vi "Controller Test Bench (6).vi"() -> ()   [LabVIEW 2022 SP3]
uses:
  <vilib>/sound2/lvsound2.llb/Sound Data Format.ctl
  <vilib>/Utility/error.llb/DialogType.ctl
  <vilib>/sound2/lvsound2.llb/Sampling Mode.ctl
  <vilib>/Analysis/4window.llb/windowTd.ctl
  <vilib>/DAQmx/read.llb/DAQmx Read (Analog 1D Wfm NChan NSamp).vi
  <vilib>/DAQmx/write.llb/DAQmx Write (Analog 1D DBL 1Chan NSamp).vi
  <vilib>/DAQmx/create/channels.llb/DAQmx Create Channel (AI-Acceleration-Accelerometer).vi
  <vilib>/DAQmx/create/channels.llb/DAQmx Create Channel (AO-Voltage-Basic).vi
  <vilib>/DAQmx/configure/timing.llb/DAQmx Timing (Sample Clock).vi
  <vilib>/DAQmx/miscellaneous.llb/DAQmx Fill In Error Info.vi
  <vilib>/measure/maspectr.llb/FFT Spectrum (Mag-Phase) for N Chan.vi
  <vilib>/DAQmx/configure/task.llb/DAQmx Configure Logging (TDMS).vi
  <vilib>/sound2/lvsound2.llb/Sound Output Set Volume (Single).vi
  <vilib>/sound2/lvsound2.llb/Sound Output Write (DBL Single).vi
  <resource>/objmgr/daqmx.rc
  <vilib>/Analysis/NI_AALPro.lvlib
  <vilib>/measure/NI_MAPro.lvlib
panel:
  out "number of samples written per channel":u32
  in  "Active Control":bool
  in  "Output Noise":bool
  in  "Log Data":bool
  out "Phase 2":cluster{"f0":dbl, "df":dbl, "phase":dbl[]}[](graph)
  out "Mag 2":cluster{"f0":dbl, "df":dbl, "magnitude":dbl[]}[](graph)
  in  "Show FFT":bool
  in  "Save FFT":bool
  in  "Start Acquisition":bool
  in  "Stop":bool
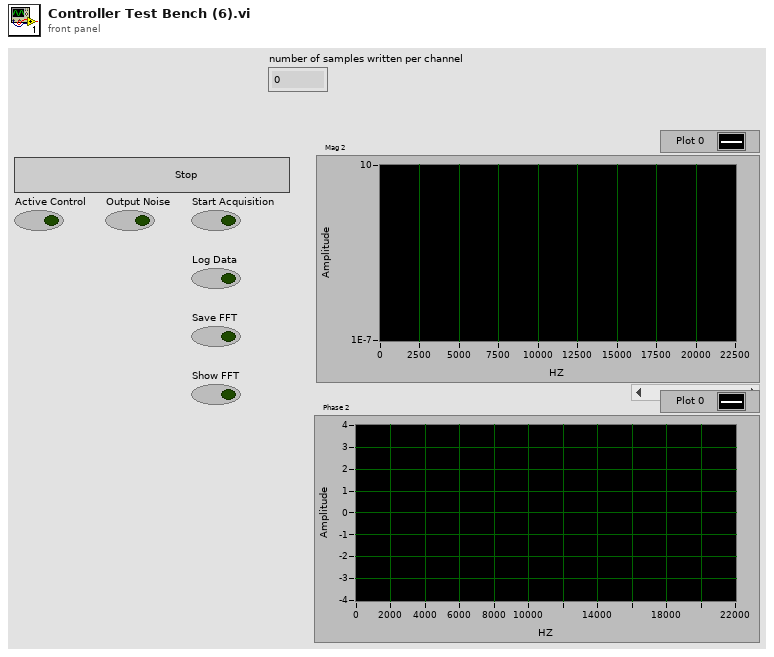
[diagram p1: front panel]
types:
  T1 = typedef "Sampling Mode.ctl" = i32
  T2 = typedef "DialogType.ctl" = u16
  T3 = typedef "Sound Data Format.ctl" = cluster{"sample rate (S/s)":dbl, "number of channels":i32, "bits per sample":i32}
  T4 = typedef "Sound Output Task ID.ctl" = u32
  T5 = typedef "NI_AALPro.lvlib/windowTd.ctl" = u32
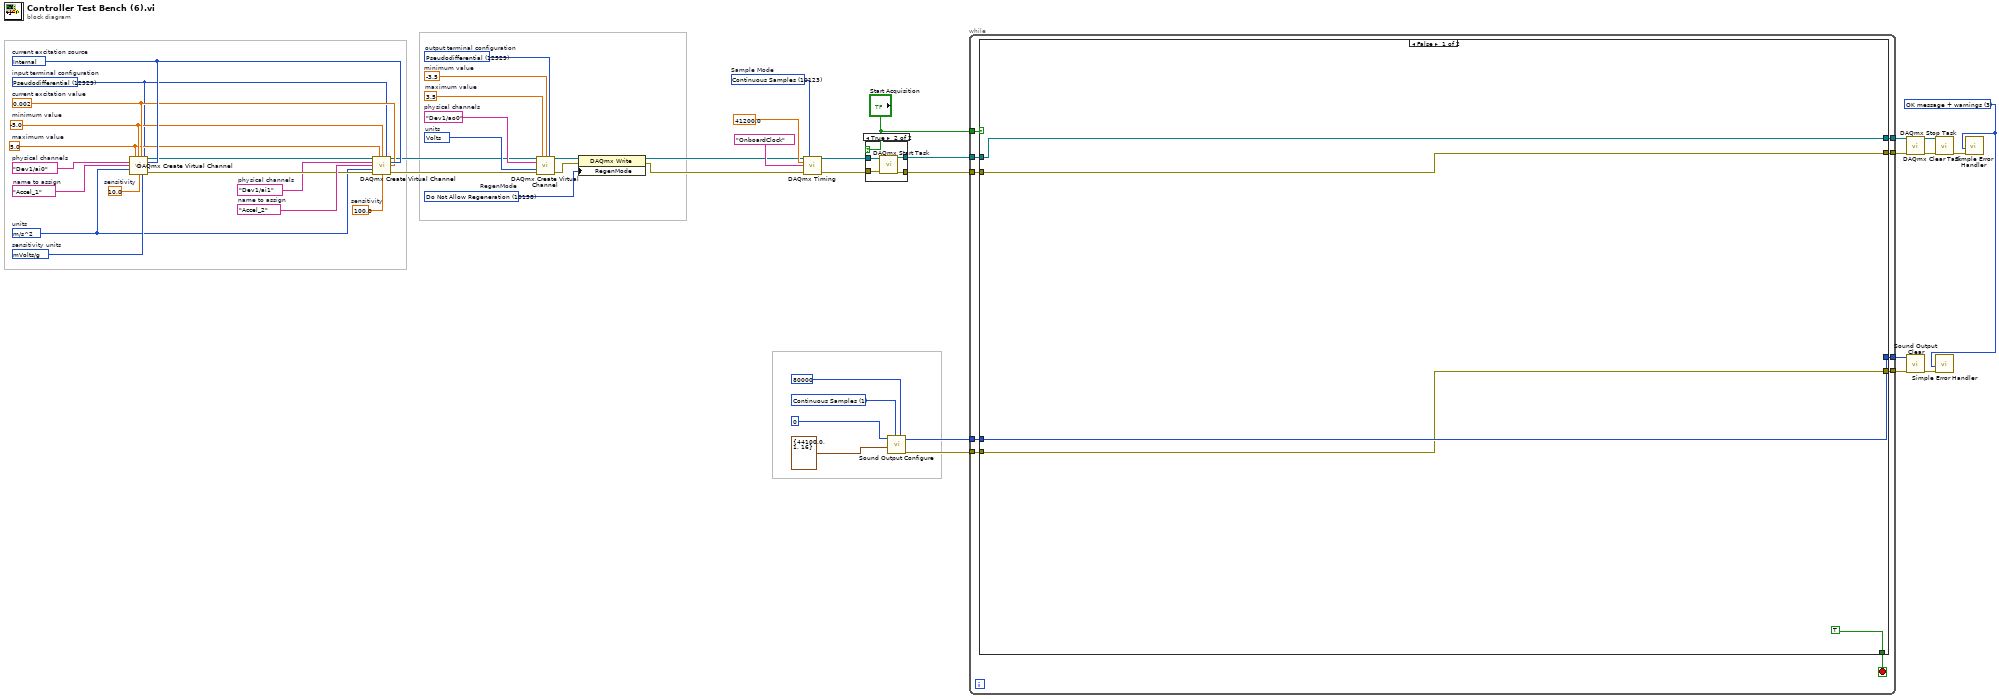
[diagram p0: block diagram]
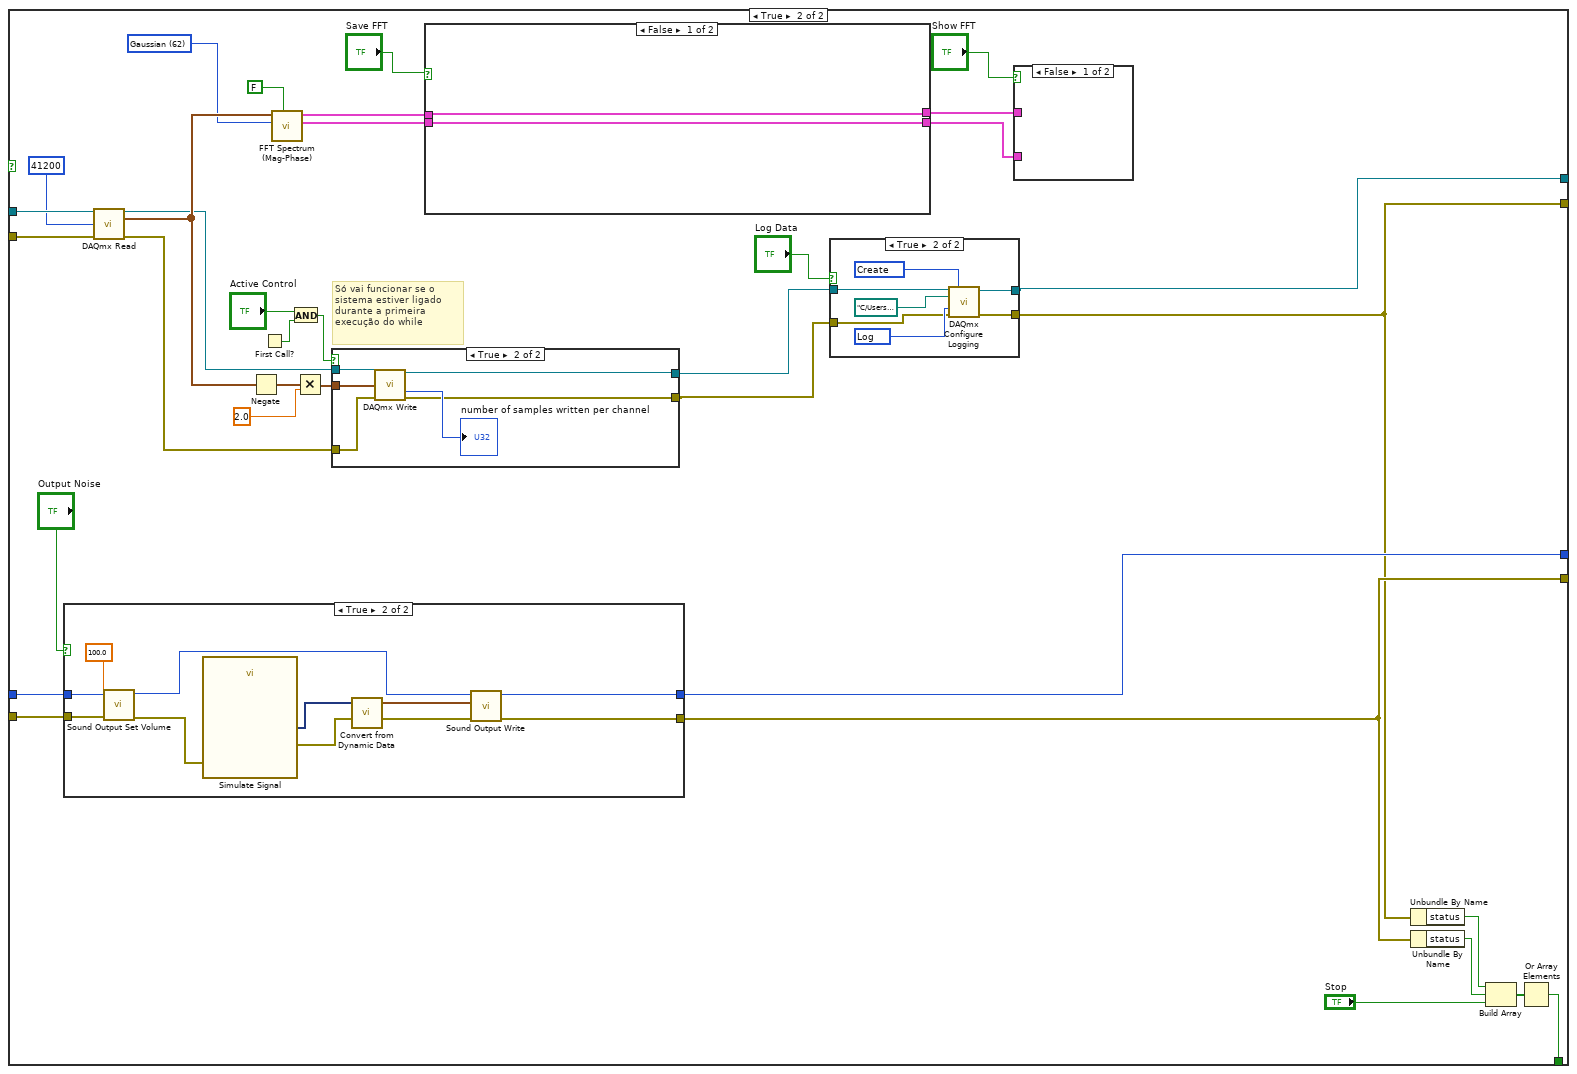
[diagram p3: hidden frame]
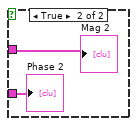
[diagram p6: hidden frame]
diagram:
  w22 = 12509 items=["mVolts/g"=12509, "Volts/g"=12510]  # sensitivity units
  w23 = 10.0  # sensitivity
  w15 = 0.002  # current excitation value
  w16 = 10200 items=["Internal"=10200, "External"=10167, "None"=10230]  # current excitation source
  w8 = tag "Dev1/ai0"  # physical channels
  w21 = 10123 items=["Finite Samples"=10178, "Continuous Samples"=10123, "Hardware Timed Single Point"=12522]  # Sample Mode
  w11 = 12529 items=["default"=-1, "RSE"=10083, "NRSE"=10078, "Differential"=10106, "Pseudodifferential"=12529]  # input terminal configuration
  w14 = -5.0  # minimum value
  w13 = 5.0  # maximum value
  w24 = "Accel_1"  # name to assign
  w12 = 12470 items=["g"=10186, "m/s^2"=12470, "in/s^2"=12471, "From Custom Scale"=10065]  # units
  w25 = 100.0  # sensitivity
  w9 = tag "Dev1/ai1"  # physical channels
  w18 = "Accel_2"  # name to assign
  w26 = T1 1 items=["Finite Samples", "Continuous Samples"] ("sample mode")
  w32 = 10158 items=["Allow Regeneration"=10097, "Do Not Allow Regeneration"=10158]  # RegenMode
  w29 = T2 3 items=["no dialog", "OK message", "continue or stop message", "OK message + warnings", "continue/stop + warnings"] ("type of dialog (OK msg:1)")
  w45 = 12529 items=["Default"=-1, "RSE"=10083, "Differential"=10106, "Pseudodifferential"=12529]  # output terminal configuration
  w46 = -3.5  # minimum value
  w47 = 3.5  # maximum value
  w43 = 10348 items=["Volts"=10348, "From Custom Scale"=10065]  # units
  w44 = tag "Dev1/ao0"  # physical channels
  n1 = call-poly <vilib>:"DAQmx Create Virtual Channel.vi"("maximum value"=w13, "minimum value"=w14, "input terminal configuration"=w11, "physical channels"=w8, "current excitation source"=w16, "name to assign"=w24, "current excitation value"=w15, "units"=w12, "sensitivity"=w23, "sensitivity units"=w22) -> ("task out"=w10:refnum<k21>, "error out"=w17:errorcluster)  [unwired: 4 in]
  n2 = call-poly <vilib>:"DAQmx Create Virtual Channel.vi"("task in"=w10, "maximum value"=w13, "minimum value"=w14, "input terminal configuration"=w11, "physical channels"=w9, "current excitation source"=w16, "name to assign"=w18, "current excitation value"=w15, "units"=w12, "error in"=w17, "sensitivity"=w25) -> ("task out"=w4:refnum<k21>, "error out"=w5:errorcluster)  [unwired: 3 in]
  n3 = call-poly <vilib>:"DAQmx Create Virtual Channel.vi"("task in"=w4, "maximum value"=w47, "minimum value"=w46, "output terminal configuration"=w45, "physical channels"=w44, "units"=w43, "error in"=w5) -> ("task out"=w31:refnum<k21>, "error out"=w3:errorcluster)  [unwired: 7 in]
  n4 = property class="DAQmx Write"(reference=w31, error in=w3, "RegenMode"=w32) -> (reference out=w1:refnum<k21>, error out=w2:errorcluster)
  n5 = call-poly <vilib>:"DAQmx Timing.vi"("task/channels in"=w1, "sample mode"=w21, "rate"=41200.0 ("Sample Rate"), "source"=tag "OnboardClock" ("Sample Clock Source"), "error in"=w2) -> ("task out"=w6:refnum<k21>, "error out"=w7:errorcluster)  [unwired: 9 in]
  n6 = case shown="True" "Start Acquisition" {
    tunnel: w7 -> [w51 w56]
    tunnel: w6 -> [w52 w55]
    tunnel: [w52 w54] -> w42
    tunnel: [w51 w53] -> w41
    frame False {
    }
    frame True {
      n7 = call <vilib>:"DAQmx Start Task.vi"("task/channels in"=w55, "error in"=w56) -> ("task out"=w54:refnum<k21>, "error out"=w53:errorcluster)  [unwired: 12 in]
    }
  }
  n8 = call <vilib>:"Sound Output Configure.vi"("number of samples/ch"=80000 ("Number of Samples/ch"), "sample mode"=w26, "sound format"=T3 {"sample rate (S/s)"=44100.0, "number of channels"=1, "bits per sample"=16} ("Sound Format"), "device ID"=u32 0 ("Device ID")) -> ("error out"=w28:errorcluster, "task ID"=w27:T4)  [unwired: 6 in]
  n9 = while {
    tunnel: w28 -> [w66]
    tunnel: w27 -> [w64]
    tunnel: w42 -> [w63]
    tunnel: w41 -> [w62]
    tunnel: [w58] -> w37
    tunnel: [w61] -> w36
    tunnel: [w59] -> w35
    tunnel: [w60] -> w34
    tunnel: "Start Acquisition" -> [w57]
    stop <- w65 stop-if-true
    n10 = case shown="False" w57 {
      tunnel: w66 -> [w68 w106]
      tunnel: [TRUE w105] -> w65
      tunnel: w64 -> [w69 w104]
      tunnel: w63 -> [w71 w103]
      tunnel: w62 -> [w70 w102]
      tunnel: [w71 w72] -> w61
      tunnel: [w69 w100] -> w60
      tunnel: [w68 w97] -> w59
      tunnel: [w70 w75] -> w58
      frame False {
      }
      frame True {
        w81 = T5 62 items=["Rectangle"=0, "Hanning"=1, "Hamming"=2, "Blackman-Harris"=3, "Exact Blackman"=4, "Blackman"=5, "Flat Top"=6, "4 Term B-Harris "=7, "7 Term B-Harris"=8, "Low Sidelobe"=9, "Blackman Nuttall"=11, "Triangle"=30, "Bartlett-Hanning"=31, "Bohman"=32, "Parzen"=33, "Welch"=34, "Kaiser"=60, "Dolph-Chebyshev"=61, "Gaussian"=62] ("window")
        # "Só vai funcionar se o sistema estiver ligado durante a primeira execução do while"
        n11 = case shown="True" "Output Noise" {
          tunnel: w106 -> [w121 w126]
          tunnel: w104 -> [w122 w127]
          tunnel: [w122 w129] -> w100
          tunnel: [w121 w128] -> w97
          frame False {
          }
          frame True {
            n12 = call-poly <vilib>:"Sound Output Set Volume.vi"("error in (no error)"=w126, "volume"=100.0, "task ID"=w127) -> ("error out"=w125:errorcluster, "task ID out"=w124:T4)  [unwired: 7 in]
            n13 = call "Simulate Signal"("error in (no error)"=w125) -> ("DC with Gaussian Noise"=w132:dynamicdata, "error out"=w131:errorcluster)  [unwired: 13 in]
            n14 = call "Convert from Dynamic Data"("Dynamic Data Type"=w132) -> ("Waveform"=w130:waveform(dbl))  [unwired: 3 in]
            n15 = call-poly <vilib>:"Sound Output Write.vi"("error in (no error)"=w131, "data"=w130, "task ID"=w124) -> ("error out"=w128:errorcluster, "task ID out"=w129:T4)  [unwired: 7 in]
          }
        }
        n16 = call-poly <vilib>:"DAQmx Read.vi"("task/channels in"=w103, "number of samples per channel"=41200, "error in"=w102) -> ("task out"=w79:refnum<k21>, "data"=w86:waveform(dbl)[], "error out"=w78:errorcluster)  [unwired: 10 in]
        n17 = Negate(x=w86) -> (-x=w87:waveform(dbl)[])
        n18 = First Call?() -> (First Call?: T/F=w89:bool)
        n19 = call-poly <vilib>:"FFT Spectrum (Mag-Phase).vi"("restart averaging (F)"=FALSE, "window"=w81, "time signals"=w86) -> ("phases"=w92:cluster{"f0":dbl, "df":dbl, "phase":dbl[]}[], "magnitudes"=w93:cluster{"f0":dbl, "df":dbl, "magnitude":dbl[]}[])  [unwired: 4 in, 3 out]
        n20 = And(x="Active Control", y=w89) -> (x .and. y?=w84:bool)
        n21 = Multiply(x=w87, y=2.0) -> (x*y=w83:waveform(dbl)[])
        n22 = case shown="True" w84 {
          tunnel: w78 -> [w108 w110]
          tunnel: [w107 w111] -> w77
          tunnel: [w108 w112] -> w76
          tunnel: w79 -> [w107 w109]
          tunnel: w83 -> [_ w114]
          frame False {
          }
          frame True {
            n23 = call-poly <vilib>:"DAQmx Write.vi"("task/channels in"=w109, "data"=w114, "error in"=w110) -> ("task out"=w111:refnum<k21>, "number of samples written per channel"=→"number of samples written per channel":u32, "error out"=w112:errorcluster)  [unwired: 10 in]
          }
        }
        n24 = case shown="False" "Save FFT" {
          tunnel: w93 -> [w115 w118]
          tunnel: w92 -> [w116 w117]
          tunnel: [w116 w117] -> w91
          tunnel: [w115 w118] -> w88
          frame False {
          }
          frame True {
          }
        }
        n25 = case shown="True" "Log Data" {
          tunnel: w77 -> [w134 w138]
          tunnel: [w134 w137] -> w72
          tunnel: w76 -> [w133 w136]
          tunnel: [w133 w135] -> w75
          frame False {
          }
          frame True {
            w139 = 15848 items=["Open"=10437, "Open or Create"=15846, "Create or Replace"=15847, "Create"=15848] ("operation")
            w140 = 15844 items=["Off"=10231, "Log"=15844, "Log and Read"=15842] ("logging mode")
            n26 = call-poly <vilib>:"DAQmx Configure Logging.vi"("task/channels in"=w138, "operation"=w139, "file path"=path "C:/Users/LAV-UFSC/Documents/LAV - TCC", "logging mode"=w140, "error in"=w136) -> ("task out"=w137:refnum<k21>, "error out"=w135:errorcluster)  [unwired: 9 in]
          }
        }
        n27 = case shown="False" "Show FFT" {
          tunnel: w88 -> [_ w120]
          tunnel: w91 -> [_ w119]
          frame False {
          }
          frame True {
            "Mag 2" <- w120
            "Phase 2" <- w119
          }
        }
        n28 = Unbundle By Name(w75) -> ("status"=w73:bool)
        n29 = Unbundle By Name(w97) -> ("status"=w74:bool)
        n30 = Build Array(w73, w74, "Stop") -> (w98:bool[])
        n31 = Or Array Elements(Boolean array=w98) -> (logical OR=w105:bool)
      }
    }
  }
  n32 = call <vilib>:"DAQmx Stop Task.vi"("task/channels in"=w36, "error in"=w37) -> ("task out"=w39:refnum<k21>, "error out"=w38:errorcluster)  [unwired: 12 in]
  n33 = call <vilib>:"Sound Output Clear.vi"("error in (no error)"=w35, "task ID"=w34) -> ("error out"=w33:errorcluster)  [unwired: 9 in]
  n34 = call <vilib>:"DAQmx Clear Task.vi"("task in"=w39, "error in"=w38) -> ("error out"=w40:errorcluster)  [unwired: 13 in]
  n35 = call <vilib>:"Simple Error Handler.vi"("type of dialog (OK msg:1)"=w29, "error in (no error)"=w33) -> ()  [unwired: 3 in, 5 out]
  n36 = call <vilib>:"Simple Error Handler.vi"("type of dialog (OK msg:1)"=w29, "error in (no error)"=w40) -> ()  [unwired: 3 in, 5 out]
